vi "derivative d Log f.vi"(6 "log T ?":bool, 7 "requested size":i32=10, 9 "temperature (min)":dbl[](array[numeric])=[1.0, 2.0, 3.0, 4.0, 5.0, 6.0, 7.0, 8.0, 9.0, 10.0], 10 "frequency (kHz)":dbl[](array[numeric])=[1.0, 2.0, 3.0, 3.0, 4.0, 5.0, 5.0, 6.0, 7.0, 8.0]) -> (3 "derivative (kHz/min)":dbl[](array[numeric])=[0.0, 1.0, 1.0, 0.0, 1.0, 1.0, 0.0, 1.0, 1.0, 1.0])   [LabVIEW 2015]
uses:
  linear interpolation - complex.vi
  <vilib>/Analysis/NI_AALBase.lvlib
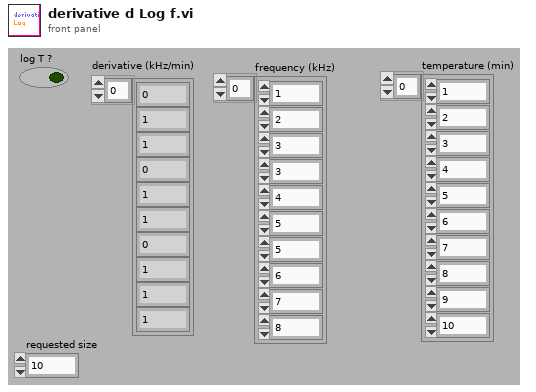
[diagram p1: front panel]
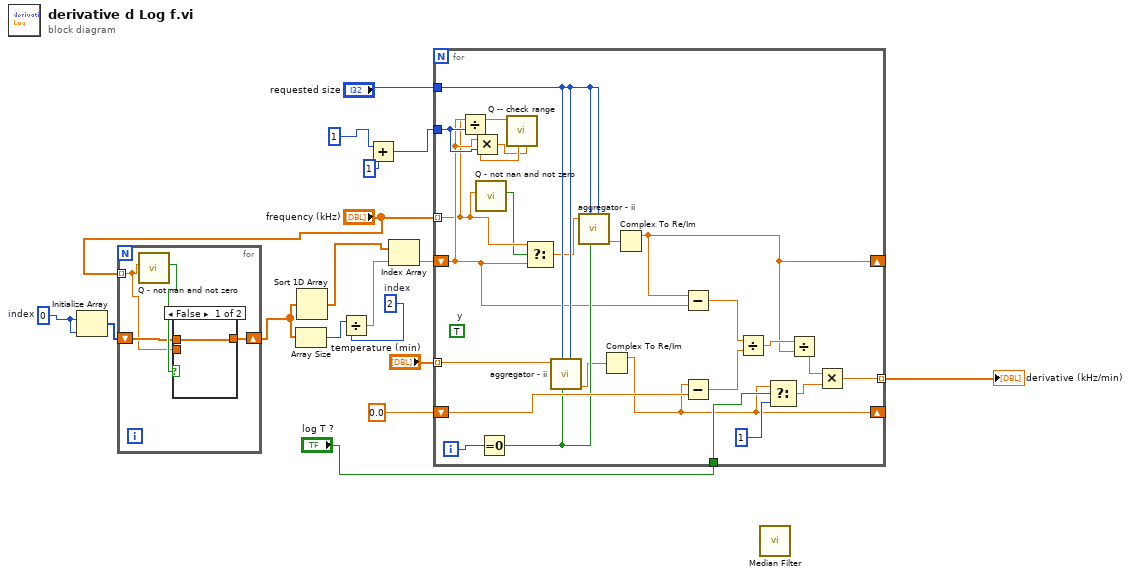
[diagram p0: block diagram]
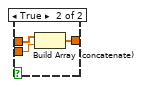
[diagram p2: hidden frame]
diagram:
  w3 = 0  # index
  w9 = 2  # index
  n1 = Initialize Array(w3, w3) -> (w1:i32[])
  n2 = for {
    tunnel: "frequency (kHz)" -> [w18] mode=indexing
    shift-right: [w20] -> w2
    shift-left: w1 -> [w19]
    n3 = call "Q - not nan and not zero.vi"("Numeric"=w18) -> ("Boolean"=w21:bool)  [unwired: 10 in]
    n4 = case shown="False" w21 {
      tunnel: [w22 w25] -> w20
      tunnel: w19 -> [w22 w24]
      tunnel: w18 -> [_ w23]
      frame False {
      }
      frame True {
        n5 = Build Array (concatenate)(w24, w23) -> (w25:dbl[])
      }
    }
  }
  n6 = Array Size(array=w2) -> (size(s)=w10:i32)
  n7 = Sort 1D Array(array=w2) -> (sorted array=w11:dbl[])
  n8 = Divide(x=w10, y=w9) -> (x/y=w8:dbl)
  n9 = Add(x=1, y=1) -> (x+y=w5:i32)
  n10 = Index Array(array=w11, index=w8) -> (element=w17:dbl)
  n11 = for {
    shift-right: [w35] -> _
    shift-left: w17 -> [w28]
    shift-right: [w33] -> _
    shift-left: 0.0 -> [w49]
    tunnel: "frequency (kHz)" -> [w27] mode=indexing
    tunnel: "temperature (min)" -> [w46] mode=indexing
    tunnel: [w40] -> w12 mode=indexing
    tunnel: "requested size" -> [w43]
    tunnel: "log T ?" -> [w37]
    tunnel: w5 -> [w32]
    i -> [w45]
    (unwired) TRUE  # y
    n12 = Divide(x=w28, y=w32) -> (x/y=w31:dbl)
    n13 = Multiply(x=w28, y=w32) -> (x*y=w30:dbl)
    n14 = call "Q - not nan and not zero.vi"("Numeric"=w27) -> ("Boolean"=w26:bool)  [unwired: 10 in]
    n15 = Equal To 0?(x=w45) -> (x = 0?=w44:bool)
    n16 = call "Q -- check range.vi"("upper"=w30, "lower"=w31, "number"=w27) -> ()  [unwired: 4 in, 5 out]
    n17 = Select(t=w27, s=w26, f=w28) -> (s? t:f=w29:dbl)
    n18 = call "aggregator - ii.vi"("requested averaging interval"=w43, "first time"=w44, "requested size"=w43, "number"=w46) -> ("interpolated average"=w34:cdb)  [unwired: 3 in, 4 out]
    n19 = call "aggregator - ii.vi"("requested averaging interval"=w43, "first time"=w44, "requested size"=w43, "number"=w29) -> ("interpolated average"=w36:cdb)  [unwired: 3 in, 4 out]
    n20 = Complex To Re/Im(x + iy=w34) -> (x=w33:dbl)  [unwired: 1 out]
    n21 = Complex To Re/Im(x + iy=w36) -> (x=w35:dbl)  [unwired: 1 out]
    n22 = Subtract(x=w35, y=w28) -> (x-y=w48:dbl)
    n23 = Subtract(x=w33, y=w49) -> (x-y=w47:dbl)
    n24 = Divide(x=w48, y=w47) -> (x/y=w42:dbl)
    n25 = Select(t=w33, s=w37, f=1) -> (s? t:f=w39:dbl)
    n26 = Divide(x=w42, y=w35) -> (x/y=w41:dbl)
    n27 = Multiply(x=w41, y=w39) -> (x*y=w40:dbl)
  }
  "derivative (kHz/min)" <- w12
  n28 = call <vilib>:"Median Filter.vi"() -> ()  [unwired: 10 in, 2 out]
